vi "Kernel - Signals Processing.vi"(7 "data in - Signals Processing":T1, 8 "error in":errorcluster, 10 "State":string, 11 "message queue":refnum<queue>) -> (0 "error out":errorcluster, 3 "message queue (out)":refnum<queue>, 4 "Stop?":bool, 5 "data out - Signals Processing":T1)   [LabVIEW 2021]
uses:
  Typedefs/Data - Signals Processing.ctl
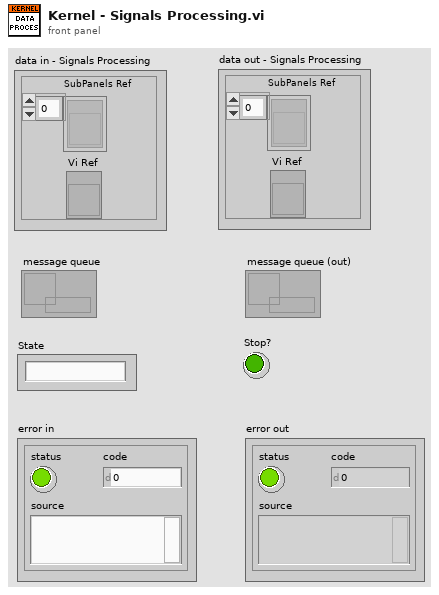
[diagram p1: front panel]
types:
  T1 = typedef "Data - Signals Processing.ctl" = cluster{"SubPanels Ref":refnum<vi>[], "Vi Ref":refnum<vi>}
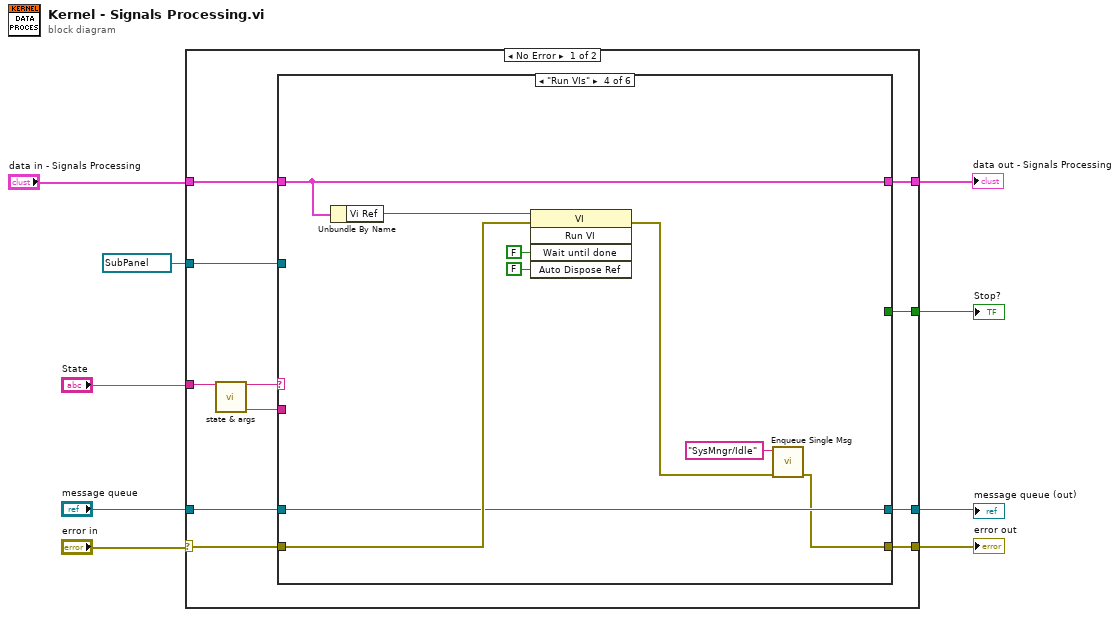
[diagram p0: block diagram]
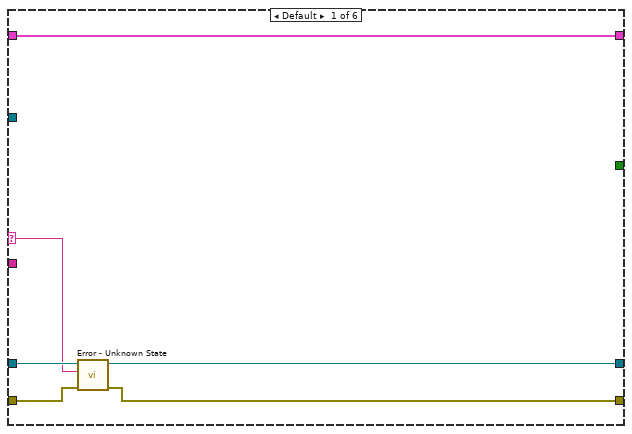
[diagram p2: hidden frame]
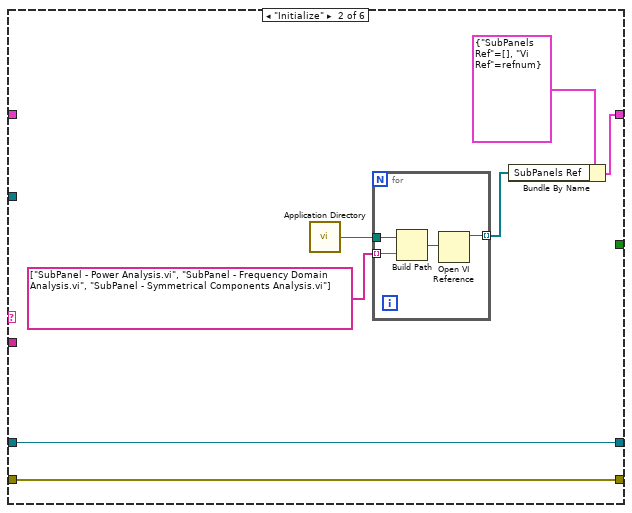
[diagram p3: hidden frame]
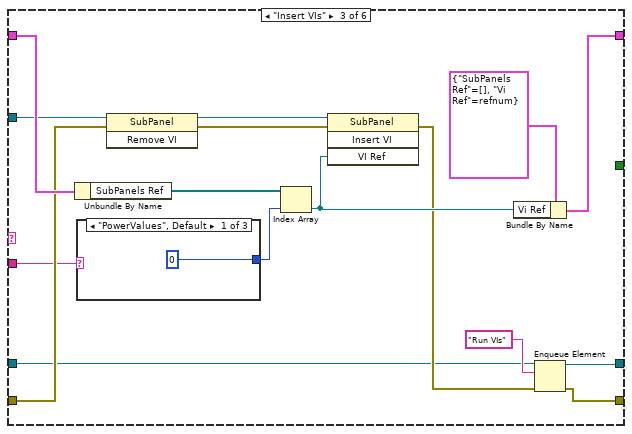
[diagram p4: hidden frame]
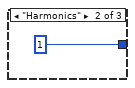
[diagram p5: hidden frame]
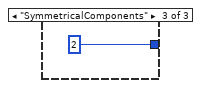
[diagram p6: hidden frame]
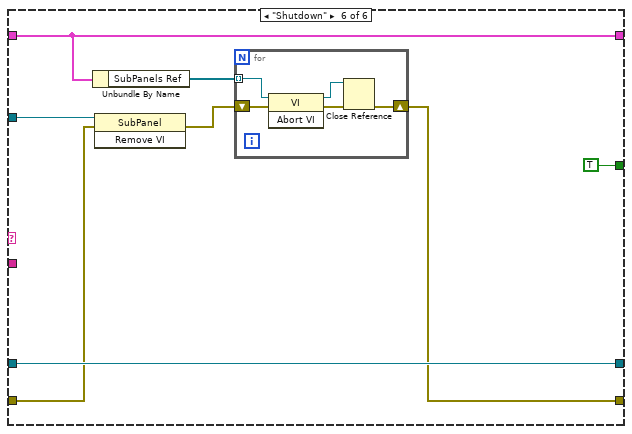
[diagram p8: hidden frame]
diagram:
  n1 = case shown="No Error" "error in" {
    selector: "error in" -> [w16 w82]
    tunnel: "State" -> [w20 _]
    tunnel: "message queue" -> [w17 w83]
    tunnel: "data in - Signals Processing" -> [w15 w84]
    tunnel: [w14 w83] -> w5
    tunnel: [w13 w82] -> w4
    tunnel: [w12 w84] -> w2
    tunnel: [w11 _] -> w6
    tunnel: refnum<vi> refnum ("reference") -> [w10 _]
    frame No Error {
      n2 = call "state & args.vi"("state:args"=w20) -> ("args"=w18:string, "state"=w19:string)  [unwired: 9 in]
      n3 = case shown="\"Run VIs\"" w19 {
        selector: w19 -> [w24 _ _ _ _ _]
        tunnel: w18 -> [_ _ w44 _ _ _]
        tunnel: w17 -> [w26 w32 w38 w60 w67 w75]
        tunnel: w16 -> [w25 w33 w46 w61 w66 w71]
        tunnel: w15 -> [w21 _ w53 w65 w68 w74]
        tunnel: [w23 w32 w40 w60 w67 w75] -> w14
        tunnel: [w22 w33 w39 w57 w66 w69] -> w13
        tunnel: [w21 w28 w49 w65 w68 w74] -> w12
        tunnel: [_ _ _ _ _ TRUE] -> w11
        tunnel: w10 -> [_ _ w48 _ _ w73]
        frame Default {
          n4 = call "Error - Unknown State.vi"("error in"=w25, "state"=w24, "queue"=w26) -> ("error out"=w22:errorcluster, "queue out"=w23:refnum<queue>)  [unwired: 7 in]
        }
        frame "Initialize" {
          n5 = call <vilib>:"Application Directory.vi"() -> ("Application Directory"=w31:path)
          n6 = for {
            tunnel: w31 -> [w36]
            tunnel: string[] ["SubPanel - Power Analysis.vi", "SubPanel - Frequency Domain Analysis.vi", "SubPanel - Symmetrical Components Analysis.vi"] -> [w35] mode=indexing
            tunnel: [w34] -> w27 mode=indexing
            n7 = Build Path(base path=w36, name or relative path=w35) -> (appended path=w37:path)
            n8 = Open VI Reference(vi path=w37) -> (vi reference=w34:refnum<vi>)  [unwired: 5 in, 1 out]
          }
          n9 = Bundle By Name(cluster=T1 {"SubPanels Ref"=[], "Vi Ref"=refnum} ("data in - Signals Processing"), "SubPanels Ref"=w27) -> (w28:T1)
        }
        frame "Insert VIs" {
          n10 = Unbundle By Name(w53) -> ("SubPanels Ref"=w52:refnum<vi>[])
          n11 = case shown="\"PowerValues\", Default" w44 {
            tunnel: [0 ("index") 1 ("index") 2 ("index")] -> w43
            frame "PowerValues", Default {
            }
            frame "Harmonics" {
            }
            frame "SymmetricalComponents" {
            }
          }
          n12 = invoke on="Invoke Node" class="SubPanel" method="Remove VI"(reference=w48, error in=w46) -> (reference out=w47:refnum<vi>, error out=w45:errorcluster)  [unwired: 1 in, 1 out]
          n13 = Index Array(array=w52, index=w43) -> (element=w51:refnum<vi>)
          n14 = invoke on="Invoke Node" class="SubPanel" method="Insert VI"(reference=w47, error in=w45, "VI Ref"=w51) -> (error out=w42:errorcluster)  [unwired: 1 in, 3 out]
          n15 = Bundle By Name(cluster=T1 {"SubPanels Ref"=[], "Vi Ref"=refnum} ("data in - Signals Processing"), "Vi Ref"=w51) -> (w49:T1)
          n16 = Enqueue Element(queue=w38, element="Run VIs", error in (no error)=w42) -> (queue out=w40:refnum<queue>, error out=w39:errorcluster)  [unwired: 1 in, 1 out]
        }
        frame "Run VIs" {
          n17 = Unbundle By Name(w65) -> ("Vi Ref"=w64:refnum<vi>)
          n18 = invoke class="VI" method="Run VI"(reference=w64, error in=w61, "Wait until done"=FALSE ("Wait Until Done"), "Auto Dispose Ref"=FALSE ("Auto Dispose Reference")) -> (error out=w58:errorcluster)  [unwired: 1 in, 4 out]
          n19 = call "Enqueue Single Msg.vi"("error in"=w58, "queue/message"="SysMngr/Idle") -> ("error out"=w57:errorcluster)  [unwired: 9 in]
        }
        frame "Error" {
        }
        frame "Shutdown" {
          n20 = Unbundle By Name(w74) -> ("SubPanels Ref"=w72:refnum<vi>[])
          n21 = invoke on="Invoke Node" class="SubPanel" method="Remove VI"(reference=w73, error in=w71) -> (error out=w70:errorcluster)  [unwired: 1 in, 2 out]
          n22 = for {
            tunnel: w72 -> [w81] mode=indexing
            shift-right: [w77] -> w69
            shift-left: w70 -> [w79]
            n23 = invoke class="VI" method="Abort VI"(reference=w81, error in=w79) -> (reference out=w80:refnum<vi>, error out=w78:errorcluster)  [unwired: 1 in, 1 out]
            n24 = Close Reference(reference=w80, error in (no error)=w78) -> (error out=w77:errorcluster)
          }
        }
      }
    }
    frame Error {
    }
  }
  "error out" <- w4
  "Stop?" <- w6
  "message queue (out)" <- w5
  "data out - Signals Processing" <- w2
